vi "Resize.vi"(10 "Capacity":u32, 11 "TypedCircularBuffer in":refnum<class "VarCircularBuffer.lvclass">) -> (3 "TypedCircularBuffer out":refnum<class "VarCircularBuffer.lvclass">)   [LabVIEW 2024, in "VarCircularBuffer.lvclass"]
uses:
  VarCircularBuffer.lvclass
  VarCircularBuffer.lvclass/VarCircularBuffer.ctl
  IsFull.vi
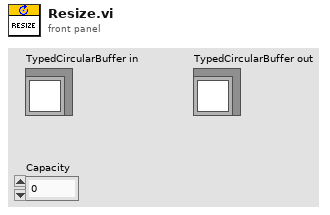
[diagram p1: front panel]
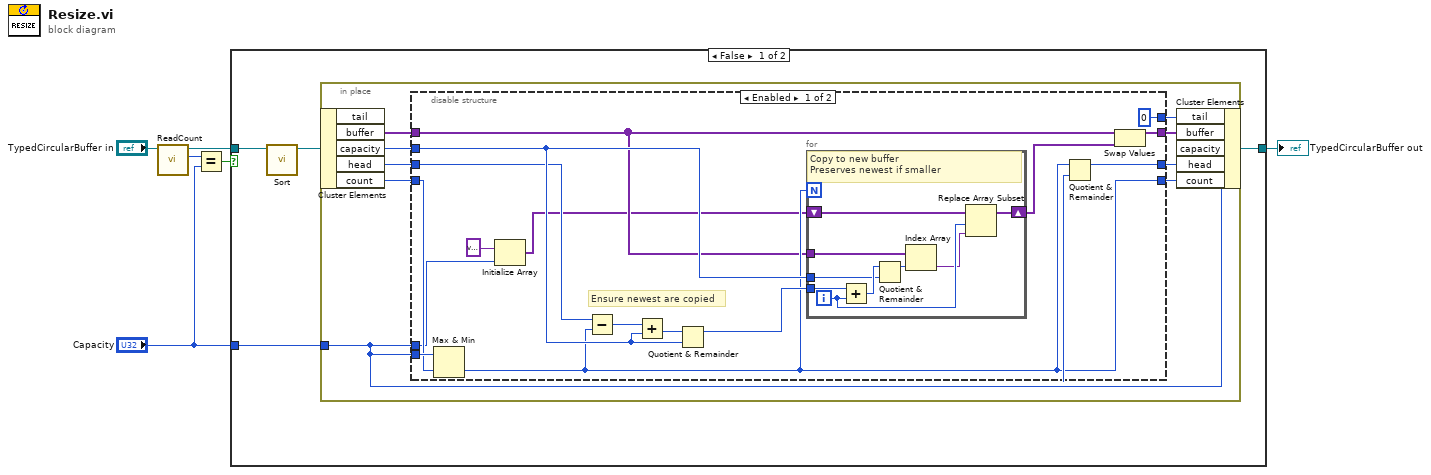
[diagram p0: block diagram]
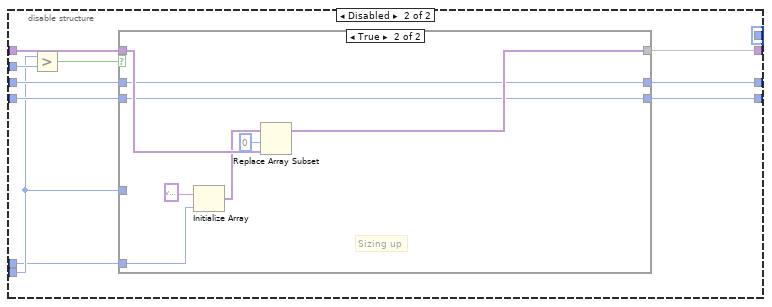
[diagram p2: hidden frame]
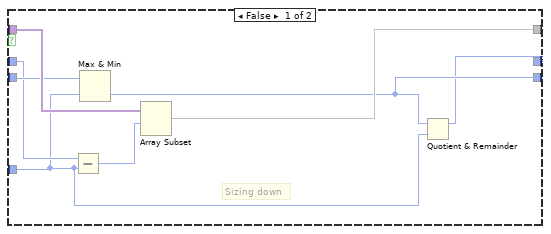
[diagram p3: hidden frame]
diagram:
  n1 = call "ReadCount.vi"("TypedCircularBuffer in"="TypedCircularBuffer in") -> ("Count"=w5:u32, "TypedCircularBuffer out"=w2:refnum<class "VarCircularBuffer.lvclass">)  [unwired: 9 in]
  n2 = Equal?(x=w5, y="Capacity") -> (x = y?=w4:bool)
  n3 = case shown="False" w4 {
    tunnel: [w9 w72] -> w3
    tunnel: w2 -> [w7 w72]
    tunnel: "Capacity" -> [w10 _]
    frame False {
      n4 = call "Sort.vi"("TypedCircularBuffer in"=w7) -> ("TypedCircularBuffer out"=w8:refnum<class "VarCircularBuffer.lvclass">)  [unwired: 10 in]
      n5 = in-place {
        in-place-border: w10 -> [w11]
        n6 = in-place-cluster #1(w8) -> ("buffer"=w13:variant[], "capacity"=w18:u32, "head"=w12:u32, "count"=w14:u32)  [unwired: 1 out]
        n7 = disable-structure shown="Enabled" {
          disable-tunnel: [w35 w51] -> w19
          disable-tunnel: w18 -> [w32 w54]
          disable-tunnel: [w30 w49] -> w17
          disable-tunnel: w11 -> [w29 w46]
          disable-tunnel: [u32 0 ("tail") u32 0 ("tail")] -> w16
          disable-tunnel: [w27 w47] -> w15
          disable-tunnel: w14 -> [w26 w48]
          disable-tunnel: w13 -> [w25 w52]
          disable-tunnel: w12 -> [w24 w50]
          disable-tunnel: w11 -> [w22 w45]
          frame Enabled {
            # "Ensure newest are copied"
            n8 = Max & Min(x=w29, y=w26) -> (min(x,y)=w27:u32)  [unwired: 1 out]
            n9 = Initialize Array(variant, w22) -> (w21:variant[])
            n10 = Subtract(x=w24, y=w27) -> (x-y=w34:u32)
            n11 = Add(x=w34, y=w32) -> (x+y=w33:u32)
            n12 = Quotient & Remainder(x=w33, y=w32) -> (x-y*floor(x/y)=w31:u32)  [unwired: 1 out]
            n13 = for {
              N: w27 -> [_]
              tunnel: w25 -> [w44]
              tunnel: w31 -> [w43]
              tunnel: w32 -> [w41]
              shift-right: [w39] -> w23
              shift-left: w21 -> [w40]
              i -> [w37]
              # "Copy to new buffer\nPreserves newest if smaller"
              n14 = Add(x=w43, y=w37) -> (x+y=w42:u32)
              n15 = Quotient & Remainder(x=w42, y=w41) -> (x-y*floor(x/y)=w38:u32)  [unwired: 1 out]
              n16 = Index Array(array=w44, index=w38) -> (element=w36:variant)
              n17 = Replace Array Subset(array=w40, new element=w36, index=w37) -> (w39:variant[])
            }
            n18 = Quotient & Remainder(x=w27, y=w29) -> (x-y*floor(x/y)=w30:u32)  [unwired: 1 out]
            n19 = Swap Values(12:w25, 14:w23) -> (1:w35:variant[])  [unwired: 1 in, 1 out]
          }
          frame Disabled {
            n20 = Greater?(x=w46, y=w54) -> (0:w53:bool)
            n21 = case shown="True" w53 {
              tunnel: w52 -> [w63 w71]
              tunnel: [w62 w70] -> w51
              tunnel: w50 -> [w60 w69]
              tunnel: [w56 w69] -> w49
              tunnel: w48 -> [w61 w68]
              tunnel: [w58 w68] -> w47
              tunnel: w46 -> [w59 _]
              tunnel: w45 -> [_ w66]
              frame False {
                # "Sizing down"
                n22 = Subtract(x=w60, y=w59) -> (x-y=w57:u32)
                n23 = Max & Min(x=w61, y=w59) -> (min(x,y)=w58:u32)  [unwired: 1 out]
                n24 = Array Subset(array=w63, index=w57) -> (w62:variant[])  [unwired: 1 in]
                n25 = Quotient & Remainder(x=w58, y=w59) -> (x-y*floor(x/y)=w56:u32)  [unwired: 1 out]
              }
              frame True {
                # "Sizing up"
                n26 = Initialize Array(variant, w66) -> (w65:variant[])
                n27 = Replace Array Subset(array=w65, new element=w71, index=0) -> (w70:variant[])
              }
            }
          }
        }
        n28 = in-place-cluster #1("tail"=w16, "buffer"=w19, "capacity"=w11, "head"=w17, "count"=w15) -> (w9:refnum<class "VarCircularBuffer.lvclass">)
      }
    }
    frame True {
    }
  }
  "TypedCircularBuffer out" <- w3
